vi "System Test.vi"(11 "Data Folder":path) -> ()   [LabVIEW 2020]
uses:
  epl-vi-lib/Signal Synthesis VIs/Controls/Multichannel (Full)/Multichannel (Full).xctl
  epl-vi-lib/Utility VIs/Type Defs/Speaker ring.ctl
  <vilib>/Analysis/5stat.llb/RMS (DBL).vi
  epl-vi-lib/Utility VIs/Math VIs/Linear to dB (scalar).vi
  epl-vi-lib/PXI DAQ VIs/DAQ Engine VIs/PXI Globals.vi
  epl-vi-lib/Signal Synthesis VIs/Waveform VIs/Noise VIs/Noise-Globals.vi
  <vilib>/Analysis/NI_AALPro.lvlib
panel:
  in  "Trigger":bool caption="Generate trigger"
  out "exit signal":bool
  out "Cal mic index":i32
  in  "Cal mic":T1={"dB SPL"=0.0, "Mode"=enum."Avg", "Mic gain (dB)"=40.0, "Sensitivity (dB V/SPL)"=-160.0} {"dB SPL" format="%.1f"}
  in  "input selections":i32[](array[numeric])
  in  "Start":bool
  out "Abort":bool
  out "AI Chans":i32[](array[numeric])
  out "AO Chans":i32[](array[numeric])
  out "AI graph":dbl[][](graph)
  in  "AO Sampling Rate (Hz)":dbl=100000.0
  in  "AI Sampling Rate (Hz)":dbl=25000.0
  in  "Total Duration (ms)":dbl=500.0
  out "Stimulus graph":dbl[][](graph)
  in  "Input Channels":i32(listbox)
  in  "Update":bool
  in  "Stop":bool
  in  "Use mapping":bool=TRUE
  in  "Quit":bool
  in  "Stimulus Channels":T2[](xcontrol)
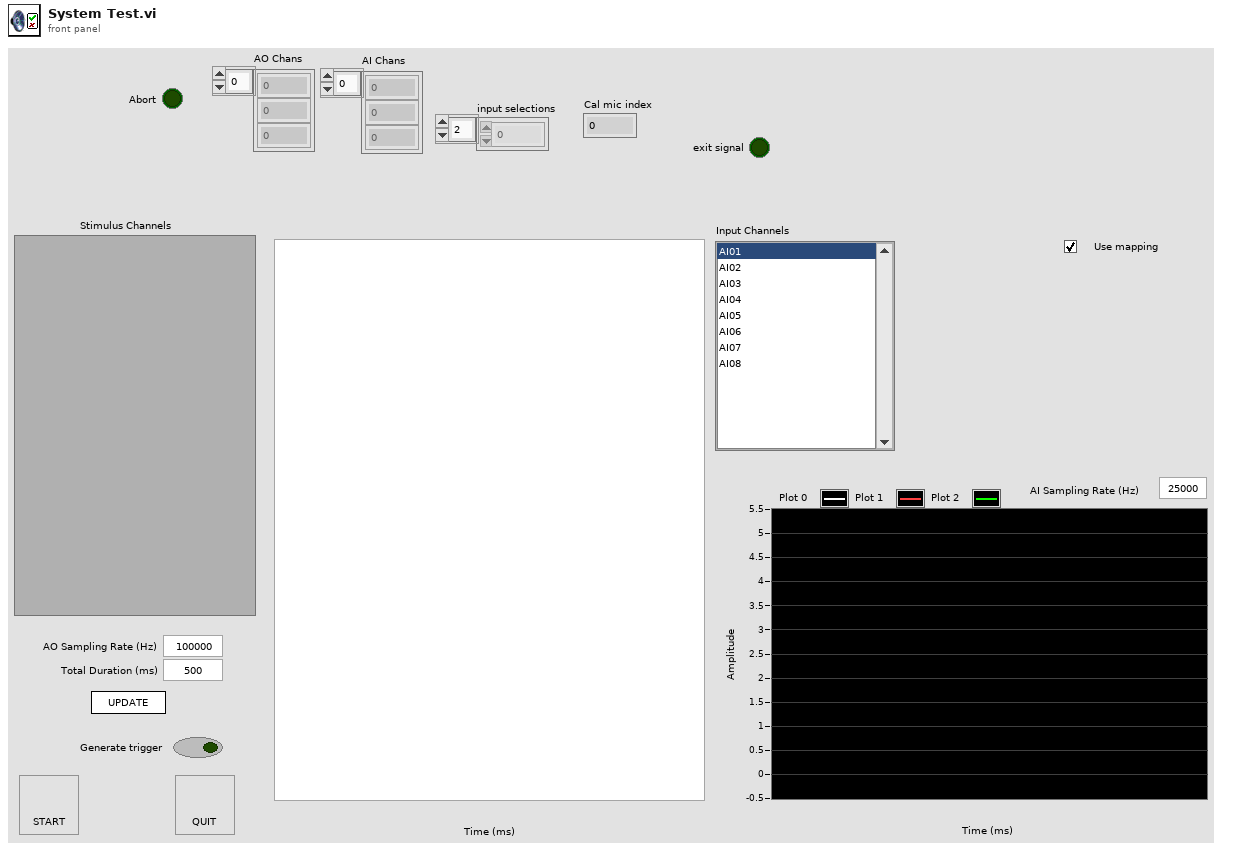
[diagram p1: front panel]
types:
  T1 = cluster{"dB SPL":dbl, "Mode":enum16{"Avg", "Peak"}, "Mic gain (dB)":dbl, "Sensitivity (dB V/SPL)":dbl}
  T2 = typedef "Stimulus Channel (Full).xctl/Full Stimulus Channel Data.ctl" = cluster{"Waveform":T3, "Filter":T20, "Burst":T22, "Level":T23, "Name":string, "Advanced":T25, "SAM":T26}
  T3 = typedef "Waveform XCtl.xctl/Waveform Data.ctl" = cluster{"Type":T4, "Tone":T5, "Pulse Train":T6, "Noise":T9, "File":T10, "FMSweep":T11, "Chirp Train":T12, "Complex Tone":cluster{"Params":T14, "Data":T16}, "Moving Ripple":T17}
  T4 = typedef "Waveform Enum.ctl" = enum16{"OFF", "Tone", "Noise", "Pulse Train", "File", "FM Sweep", "Chirp Train", "Complex Tone", "FM Tone", "Moving Ripple"}
  T5 = typedef "Tone Params.ctl" = cluster{"Frequency (kHz)":dbl, "Last Freq":dbl, "Last Phase":dbl}
  T6 = typedef "Pulse Train Params.ctl" = cluster{"Pulse width (us)":dbl, "Pulse rate (Hz)":dbl, "Gap (ms)":dbl, "Polarity":T7, "PT State":T8, "Asynch":bool}
  T7 = typedef "Pulse Polarity.ctl" = enum16{"POS", "NEG", "POS-NEG", "NEG-POS"}
  T8 = typedef "PT-Continuous State.ctl" = cluster{"Template":dbl[], "Nperiod":i32, "Index":i32, "Pulse Rate (Hz)":dbl, "Phase (cycles)":dbl, "Noff":i32}
  T9 = typedef "Noise Params.ctl" = cluster{"InvFilt":bool, "Noise":dbl[], "CurPt":i32, "Aweight":bool, "Seed":i32, "afile":path}
  T10 = typedef "StimFile-Params.ctl" = cluster{"Filename":path, "Signal":dbl[], "Channel":i32, "stream":bool, "offset":i32, "nreps":i32, "loops":i32, "Randomize":bool, "order":i32[], "Seed":i32, "Tokens":i32}
  T11 = typedef "FM Sweep Params.ctl" = cluster{"Rate (oct/s)":dbl, "Fmin (Hz)":dbl, "Fmax (Hz)":dbl, "Ramp (ms)":dbl, "Linear":bool}
  T12 = typedef "Chirp Train.ctl" = cluster{"Params":T13, "Data":cluster{"WF":dbl[]}}
  T13 = typedef "Chirp Train Params.ctl" = cluster{"Fmin (kHz)":dbl, "Fmax (kHz)":dbl, "Compensate":bool, "Duration (ms)":dbl}
  T14 = typedef "CT-Params.ctl" = cluster{"F0 (Hz)":dbl, "Band":cluster{"Flow (Hz)":dbl, "Fhigh (Hz)":dbl}, "Phase":T15, "Min F0 (Hz)":dbl, "Max F0 (Hz)":dbl, "ContinRandPhase":bool, "Max peak factor":dbl, "Max mod depth":dbl, "MinHarmNum":i32, "MaxHarmNum":i32, "Level Mode":enum16{"per component", "overall rms"}, "% jitter":dbl}
  T15 = typedef "CT-Phase Enum.ctl" = enum16{"Cosine", "Random", "Alternating"}
  T16 = typedef "CT-Runtime Data.ctl" = cluster{"Ncomp":i32, "MinHarm":i32, "Phase":dbl[], "Amplitude":dbl[], "Npts/frame":i32, "Last F0":dbl, "Fmin":dbl, "Fmax":dbl, "Lslope":dbl, "randphase":bool, "overall rms":bool, "fmult":dbl[], "jittered":bool}
  T17 = typedef "Moving Ripple.ctl" = cluster{"Params":T18, "Data":T19}
  T18 = typedef "Moving Ripple.Params.ctl" = cluster{"Fmin":dbl, "Fmax":dbl, "Density":dbl, "Velocity":dbl, "Depth":dbl, "Phase":dbl, "Comp/oct":i32}
  T19 = typedef "Moving Ripple.Data.ctl" = cluster{"Freq":dbl[], "A":dbl[], "phase":dbl[], "Phase":dbl}
  T20 = typedef "Advanced Filter XCtl.xctl/Filter Data.ctl" = cluster{"Type":enum16{"Lowpass", "Highpass", "Bandpass", "Bandstop", "OFF"}, "CF (kHz)":dbl, "BW (kHz)":dbl, "Cascade":bool, "Quadrature":bool, "Scale Factor":dbl, "Stages":cluster{"IIR Filter":cluster{"filter structure":enum32{"IIR 2nd Order", "IIR 4th Order"}, "Reverse Coefficients":dbl[], "Forward Coefficients":dbl[]}, "State":dbl[]}[], "Class":enum16{"Elliptic", "Butterworth"}, "Order":i32, "BWUnits":T21}
  T21 = typedef "Filter-Bandwidth Units.ctl" = enum16{"Linear", "Octaves", "Min-Max"}
  T22 = typedef "Burst Control.xctl/Burst Data.ctl" = cluster{"Active":bool, "Delay (ms)":dbl, "Duration (ms)":dbl, "Ramp (ms)":dbl, "Rate (Hz)":dbl, "Trepeat (ms)":dbl, "Repeat":bool}
  T23 = typedef "Level XCtl.xctl/Level Data.ctl" = cluster{"Level":dbl, "Units":T24, "Max":dbl, "Multiplier":dbl, "Cal File":path, "Cal":cluster{"Freq (Hz)":dbl[], "Mag (dB SPL)":dbl[], "Phase (deg)":dbl[]}}
  T24 = typedef "Level Units.ctl" = enum16{"dB atten", "dB SPL", "dB re 1 Vrms", "dB V/Hz½", "mW", "dB HL", "Volts", "dB mW"}
  T25 = typedef "Advanced Stimulus Options.xctl/Advanced Stimulus Options.ctl" = cluster{"Rep Mask":string, "AltPol":bool, "Var":string, "Expr":string, "Persist":bool}
  T26 = typedef "SAM Params.ctl" = cluster{"Active":bool, "Frequency (Hz)":dbl, "Depth":dbl, "Init Phase (cycles)":dbl, "phase (degrees)":dbl, "Asynch":bool}
  T27 = typedef "Multichannel (Full).xctl/Data.ctl" = T2[]
  T28 = typedef "Speaker ring.ctl" = enum16{"Right primary", "Right secondary", "Left primary", "Left secondary"}
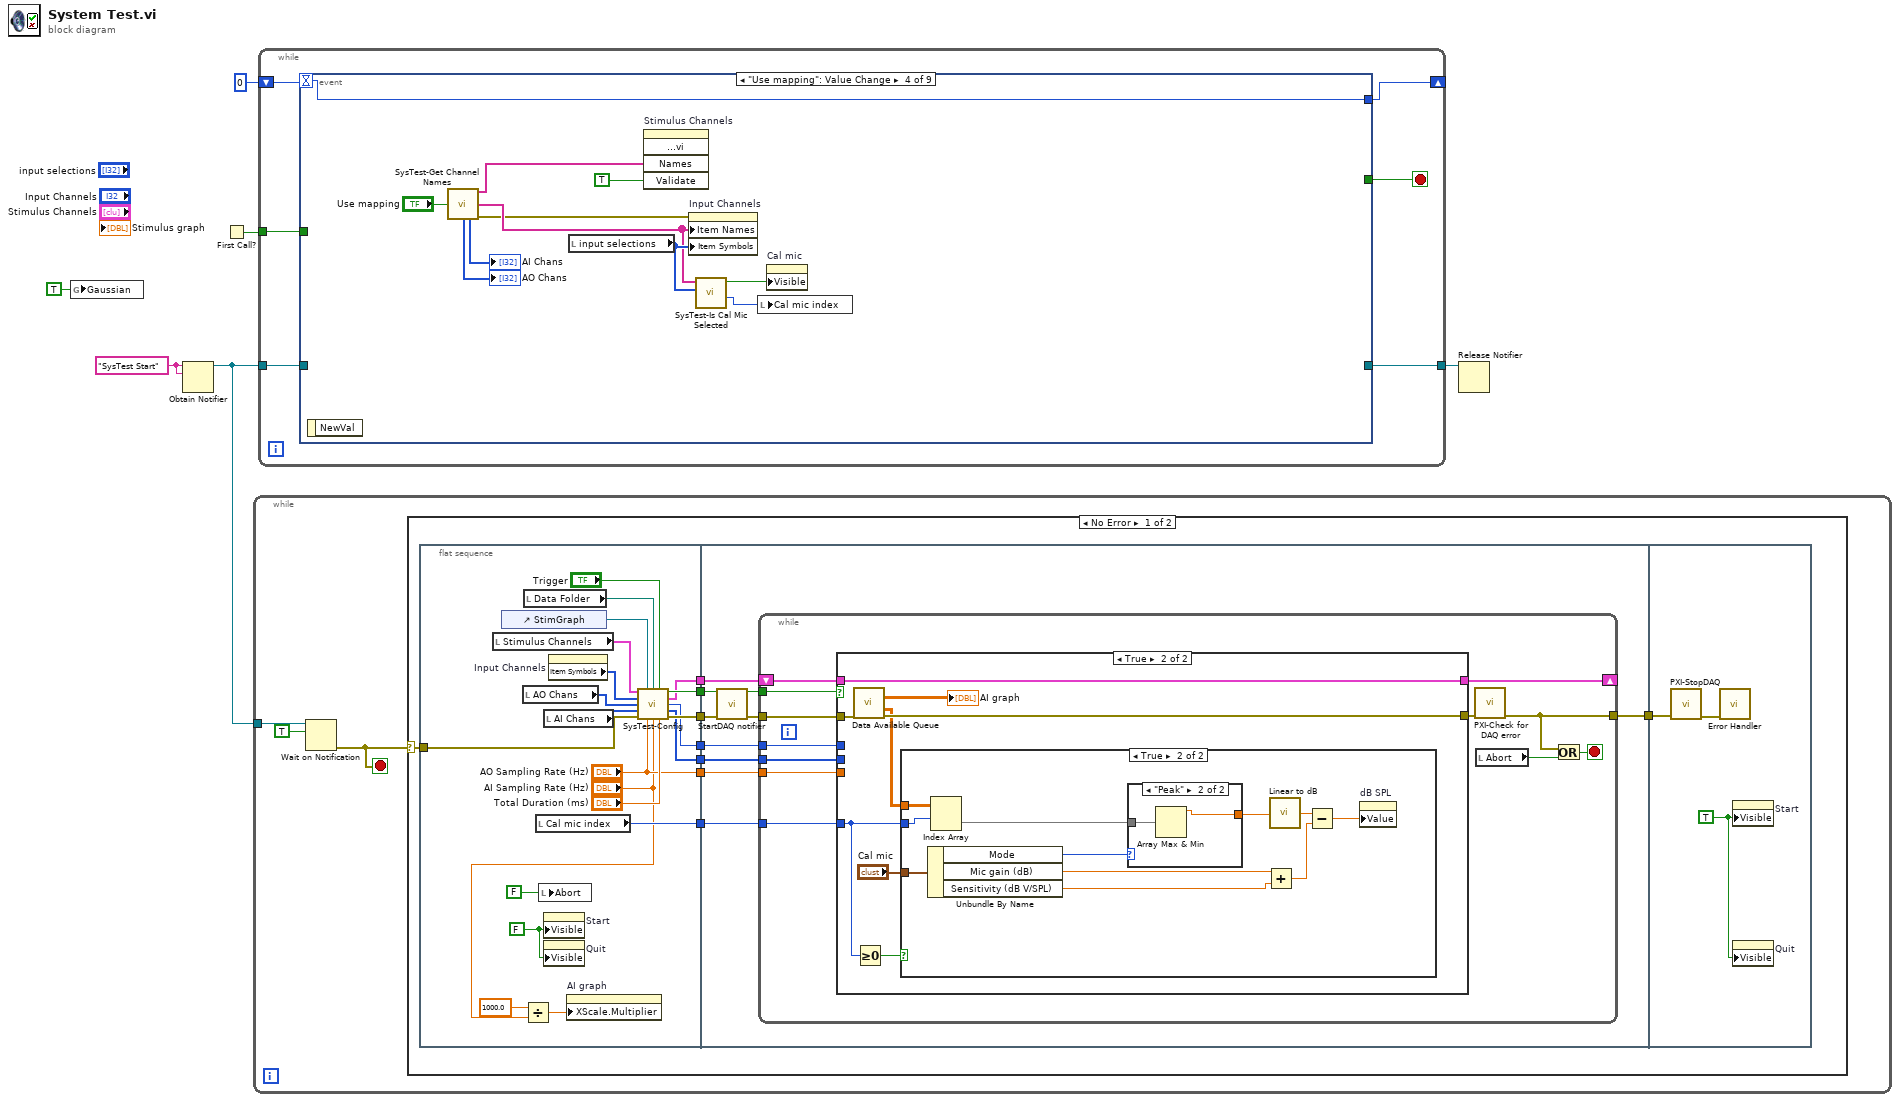
[diagram p0: block diagram]
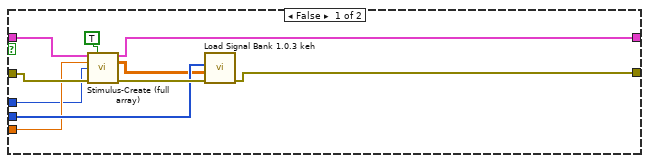
[diagram p2: hidden frame]
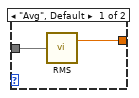
[diagram p4: hidden frame]
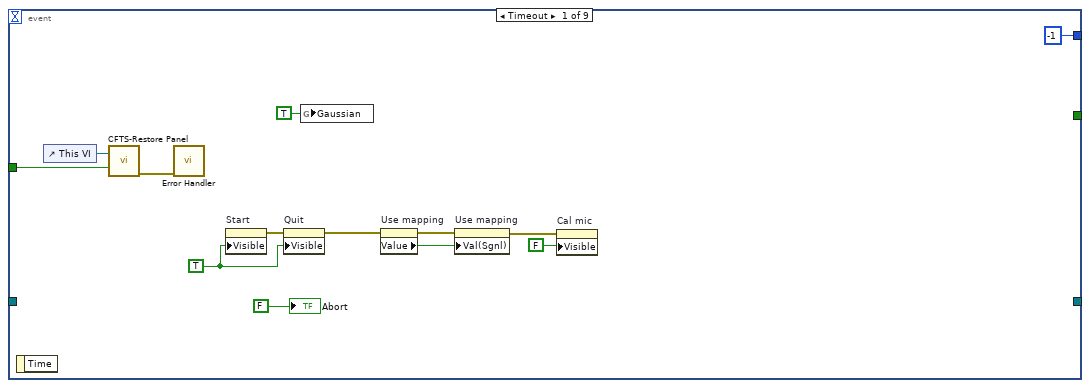
[diagram p6: hidden frame]
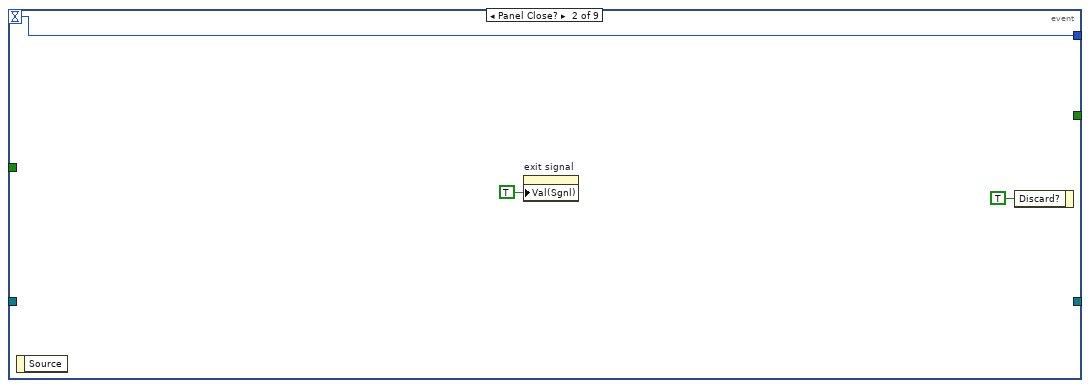
[diagram p7: hidden frame]
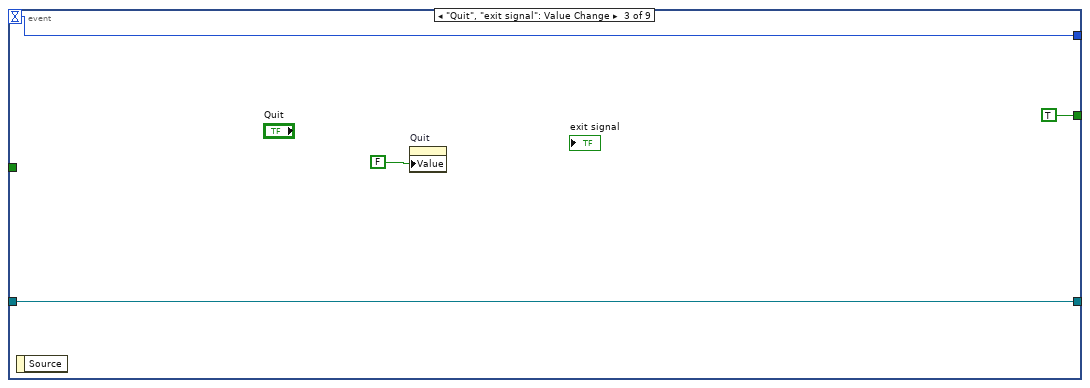
[diagram p8: hidden frame]
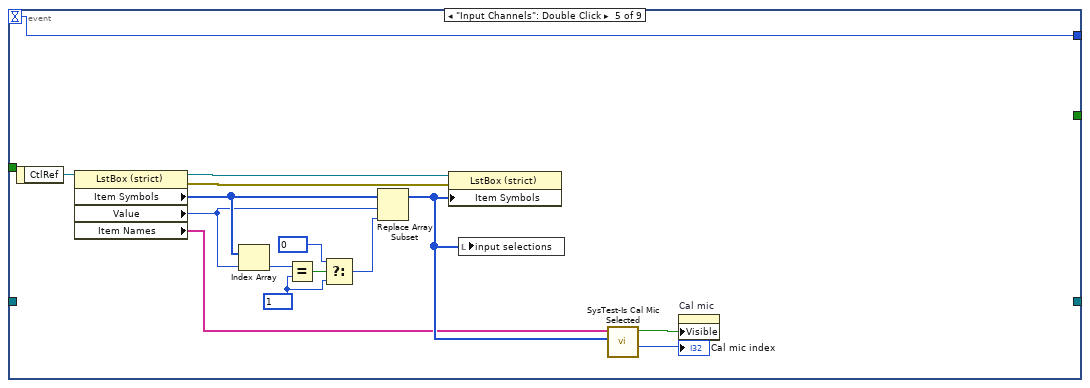
[diagram p9: hidden frame]
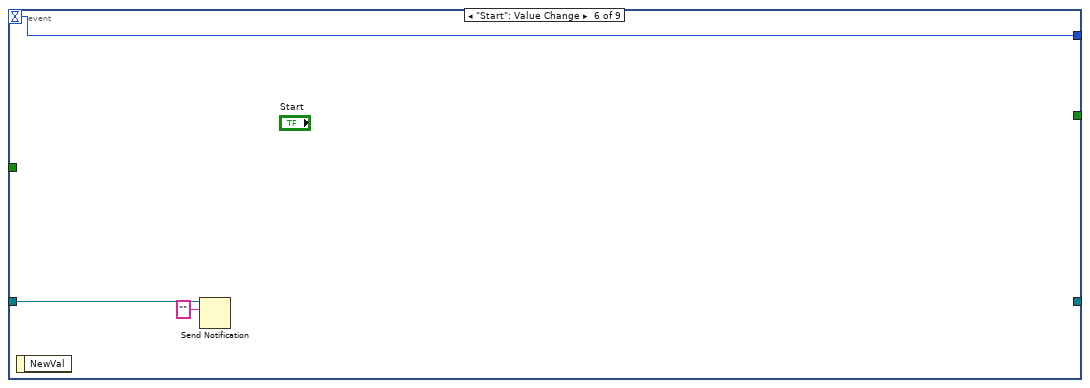
[diagram p10: hidden frame]
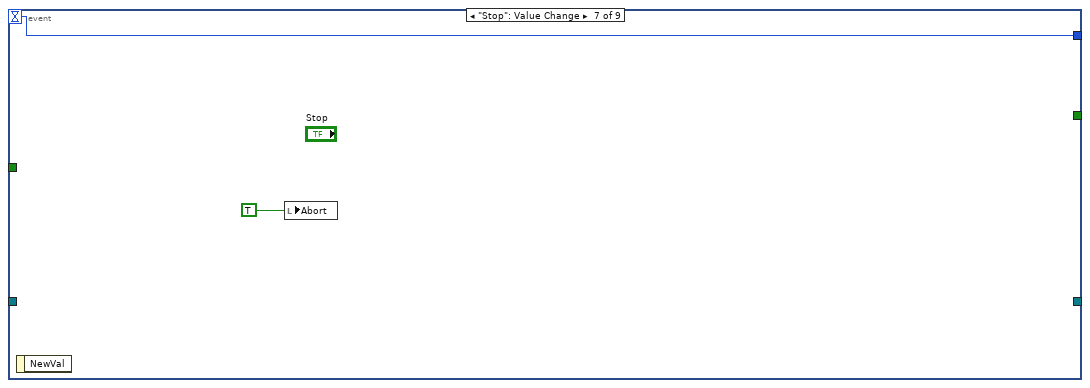
[diagram p11: hidden frame]
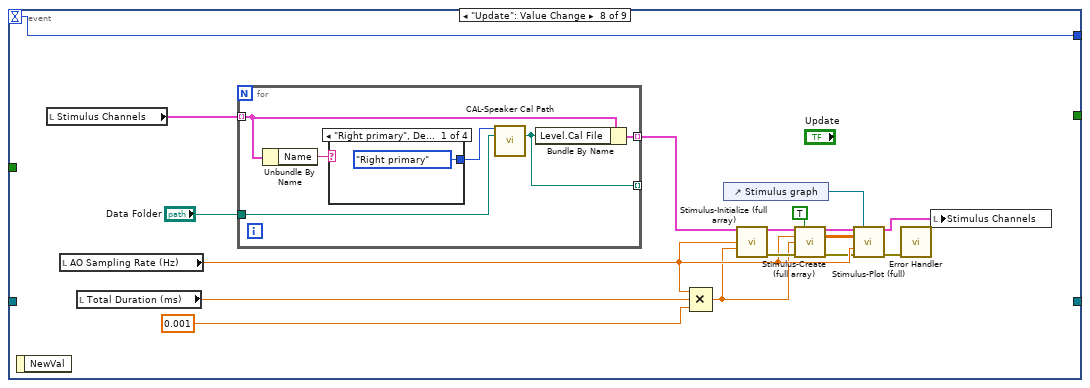
[diagram p12: hidden frame]
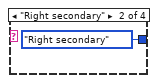
[diagram p13: hidden frame]
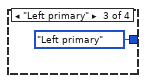
[diagram p14: hidden frame]
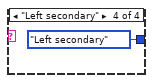
[diagram p15: hidden frame]
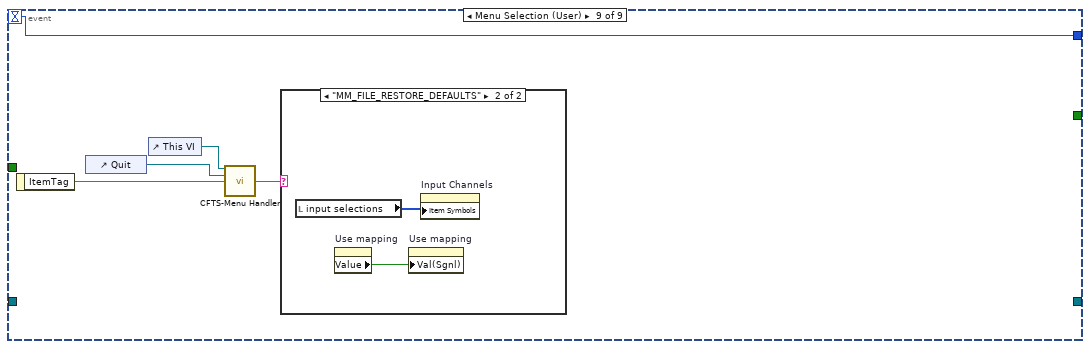
[diagram p16: hidden frame]
diagram:
  w5 = "SysTest Start" ("name (unnamed)")
  n1 = global write "Noise-Globals.vi" "Gaussian"(TRUE ("Gaussian")) -> ()
  n2 = Obtain Notifier(name (unnamed)=w5, notification data type=w5) -> (notifier out=w6:refnum<notifier>)  [unwired: 2 in, 2 out]
  n3 = First Call?() -> (First Call?: T/F=w2:bool)
  n4 = while {
    tunnel: w6 -> [w9]
    stop <- w7 stop-if-true
    n5 = Wait on Notification(notifier=w9, ignore previous (F)=TRUE) -> (error out=w7:errorcluster)  [unwired: 2 in, 3 out]
    n6 = case shown="No Error" w7 {
      selector: w7 -> [w18 _]
      frame No Error {
        n7 = flat-sequence {
          tunnel: w18 -> [w36]
          tunnel: [w34] -> w17
          tunnel: [w31] -> w15
          tunnel: [w27] -> w14
          tunnel: [w26] -> w13
          tunnel: ["AO Sampling Rate (Hz)"] -> w12
          tunnel: [w24] -> w11
          tunnel: [w23] -> w10
          tunnel: w17 -> [w48]
          tunnel: [w47] -> w16
          tunnel: w15 -> [w45]
          tunnel: w14 -> [w44]
          tunnel: w13 -> [w43]
          tunnel: w12 -> [w42]
          tunnel: w11 -> [w41]
          tunnel: w10 -> [w40]
          tunnel: w16 -> [w96]
          frame #0 {
            w30 = FALSE ("Visible")
            n8 = local read "Stimulus Channels"() -> (w39:T2[])
            n9 = control-ref of="StimGraph"() -> (w32:refnum<vi>)
            n10 = local read "AO Chans"() -> (w38:i32[])
            n11 = Divide(x=1000.0, y="AI Sampling Rate (Hz)") -> (x/y=w21:dbl)
            n12 = local read "Data Folder"() -> (w28:path)
            n13 = local read "Cal mic index"() -> (w27:i32)
            n14 = local write "Abort"(FALSE ("Global Abort")) -> ()
            n15 = local read "AI Chans"() -> (w37:i32[])
            n16 = property on="Start" class="Bool"("Visible"=w30) -> ()  [unwired: 2 in, 2 out]
            n17 = property on="Quit" class="Bool (strict)"("Visible"=w30) -> ()  [unwired: 2 in, 2 out]
            n18 = property on="Input Channels" class="LstBox (strict)"() -> ("Item Symbols"=w33:i32[])  [unwired: 2 in, 2 out]
            n19 = property on="AI graph" class="WFGraph (strict)"("XScale.Multiplier"=w21) -> ()  [unwired: 2 in, 2 out]
            n20 = call "SysTest-Config.vi"("AO Control"=w39, "Waveform Graph"=w32, "Data Folder"=w28, "Trigger"="Trigger", "Item Symbols"=w33, "AO Chans"=w38, "AI Chans"=w37, "error in (no error)"=w36, "AO Sampling Rate (Hz)"="AO Sampling Rate (Hz)", "AI Sampling Rate (Hz)"="AI Sampling Rate (Hz)", "Total Duration (ms)"="Total Duration (ms)") -> ("have AI?"=w31:bool, "StimChans Out"=w24:T27, "AO npts"=w23:i32, "AO Chans"=w26:i32[], "error out"=w34:errorcluster)
          }
          frame #1 {
            n21 = call "StartDAQ notifier.vi"("error in (no error)"=w48) -> ("error out"=w46:errorcluster)  [unwired: 6 in]
            n22 = while {
              tunnel: w46 -> [w60]
              tunnel: [w54] -> w47
              tunnel: w45 -> [w57]
              tunnel: w44 -> [w55]
              tunnel: w43 -> [w53]
              shift-right: [w52] -> _
              shift-left: w41 -> [w51]
              tunnel: w42 -> [w50]
              tunnel: w40 -> [w49]
              stop <- w59 stop-if-true
              n23 = case shown="True" w57 {
                tunnel: w60 -> [w70 w78]
                tunnel: [w62 w77] -> w58
                tunnel: w55 -> [_ w75]
                tunnel: w53 -> [w67 _]
                tunnel: [w65 w72] -> w52
                tunnel: w51 -> [w64 w72]
                tunnel: w50 -> [w63 _]
                tunnel: w49 -> [w61 _]
                frame False {
                  n24 = call "Stimulus-Create (full array).vi"("StimChan"=w64, "Apply multipliers? (F)"=TRUE ("Apply multipliers?"), "Sampling Rate (Hz)"=w63, "Npts"=w61, "error in (no error)"=w70) -> ("StimChan Out"=w65:T2[], "Waveform"=w66:dbl[][], "error out"=w68:errorcluster)  [unwired: 7 in, 1 out]
                  n25 = call "Load Signal Bank 1.0.3 keh.vi"("error in (no error)"=w68, "Input array"=w66, "Active AO Array"=w67) -> ("error out"=w62:errorcluster)  [unwired: 6 in, 2 out]
                }
                frame True {
                  n26 = call "Data Available Queue.vi"("error in (no error)"=w78) -> ("Waveform Graph"=→"AI graph":dbl[][], "AI Waveforms"=w74:dbl[][], "error out"=w77:errorcluster)  [unwired: 10 in, 2 out]
                  n27 = Greater Or Equal To 0?(x=w75) -> (x >= 0?=w76:bool)
                  n28 = case shown="True" w76 {
                    tunnel: w75 -> [_ w88]
                    tunnel: w74 -> [_ w89]
                    tunnel: "Cal mic" -> [_ w81]
                    frame False {
                    }
                    frame True {
                      n29 = Unbundle By Name(w81) -> ("Mode"=w80:enum16{"Avg", "Peak"}, "Mic gain (dB)"=w87:dbl, "Sensitivity (dB V/SPL)"=w86:dbl)
                      n30 = Index Array(array=w89, index (row)=w88) -> (element=w83:dbl[])  [unwired: 1 in]
                      n31 = case shown="\"Peak\"" w80 {
                        tunnel: [w91 w92] -> w84
                        tunnel: w83 -> [w90 w93]
                        frame "Avg", Default {
                          n32 = call-poly <vilib>:"RMS.vi"("X"=w90) -> ("rms value"=w91:dbl)  [unwired: 1 out]
                        }
                        frame "Peak" {
                          n33 = Array Max & Min(array=w93) -> (max value=w92:dbl)  [unwired: 3 out]
                        }
                      }
                      n34 = Add(x=w87, y=w86) -> (x+y=w82:dbl)
                      n35 = call-poly "Linear to dB.vi"("Linear"=w84) -> ("dB"=w85:dbl)
                      n36 = Subtract(x=w85, y=w82) -> (x-y=w79:dbl)
                      n37 = property on="dB SPL" class="DigNum (strict)"("Value"=w79) -> ()  [unwired: 2 in, 2 out]
                    }
                  }
                }
              }
              n38 = call "PXI-Check for DAQ error.vi"("error in (no error)"=w58) -> ("error out"=w54:errorcluster)  [unwired: 14 in]
              n39 = local read "Abort"() -> (w56:bool)
              n40 = Or(x=w54, y=w56) -> (x .or. y?=w59:bool)
            }
          }
          frame #2 {
            w94 = TRUE ("Visible")
            n41 = call "PXI-StopDAQ.vi"("error in (no error)"=w96) -> ("error out"=w95:errorcluster)  [unwired: 6 in]
            n42 = call "Error Handler.vi"("error in (no error)"=w95) -> ()  [unwired: 13 in, 2 out]
            n43 = property on="Start" class="Bool"("Visible"=w94) -> ()  [unwired: 2 in, 2 out]
            n44 = property on="Quit" class="Bool (strict)"("Visible"=w94) -> ()  [unwired: 2 in, 2 out]
          }
        }
      }
      frame Error {
      }
    }
  }
  n45 = while {
    tunnel: w6 -> [w101]
    tunnel: [w100] -> w4
    shift-right: [w98] -> _
    shift-left: 0 -> [w99]
    tunnel: w2 -> [w97]
    stop <- w102 stop-if-true
    n46 = event shown="[3] \"Use mapping\": Value Change" {
      selector: _ -> [_ _ _ _ _ _ _ _ _]
      dyn-events: _ -> [_ _ _ _ _ _ _ _ _]
      timeout: w99 -> [_ w116 w120 w132 w138 w149 w152 w170 w182]
      tunnel: [_ _ TRUE _ _ _ _ _ _] -> w102
      tunnel: w101 -> [_ _ w121 _ _ w151 _ _ _]
      tunnel: [_ _ w121 _ _ _ _ _ _] -> w100
      tunnel: [-1 w116 w120 w132 w138 w149 w152 w170 w182] -> w98
      tunnel: w97 -> [w110 _ _ _ _ _ _ _ _]
      event Timeout {
        w113 = TRUE ("Visible")
        n47 = event-data() -> ()  [unwired: 1 in, 1 out]
        n48 = control-ref of="This VI"() -> (w111:refnum<vi>)
        n49 = call "CFTS-Restore Panel.vi"("VI refnum"=w111, "Restore?"=w110) -> ("error out"=w104:errorcluster)  [unwired: 12 in, 1 out]
        n50 = call "Error Handler.vi"("error in (no error)"=w104) -> ()  [unwired: 13 in, 2 out]
        n51 = property on="Start" class="Bool"("Visible"=w113) -> (error out=w114:errorcluster)  [unwired: 2 in, 1 out]
        n52 = property on="Quit" class="Bool (strict)"(error in=w114, "Visible"=w113) -> (error out=w109:errorcluster)  [unwired: 1 in, 1 out]
        n53 = global write "Noise-Globals.vi" "Gaussian"(TRUE ("Gaussian")) -> ()
        n54 = property on="Use mapping" class="Bool (strict)"(error in=w109) -> (error out=w107:errorcluster, "Value"=w108:bool)  [unwired: 1 in, 1 out]
        n55 = property on="Use mapping" class="Bool (strict)"(error in=w107, "Val(Sgnl)"=w108) -> (error out=w106:errorcluster)  [unwired: 1 in, 1 out]
        n56 = property on="Cal mic" class="Clust (strict)"(error in=w106, "Visible"=FALSE) -> ()  [unwired: 1 in, 2 out]
        "Abort" <- FALSE ("quitting?")
      }
      event Panel Close? {
        n57 = event-data() -> ()  [unwired: 1 in, 1 out]
        n58 = property on="exit signal" class="Bool (strict)"("Val(Sgnl)"=TRUE ("Value (Signaling)")) -> ()  [unwired: 2 in, 2 out]
        n59 = event-data("Discard?"=TRUE) -> ()  [unwired: 1 in, 1 out]
      }
      event "Quit", "exit signal": Value Change {
        n60 = event-data() -> ()  [unwired: 1 in, 1 out]
        n61 = property on="Quit" class="Bool (strict)"("Value"=FALSE) -> ()  [unwired: 2 in, 2 out]
      }
      event "Use mapping": Value Change {
        n62 = event-data() -> ()  [unwired: 1 in, 1 out]
        n63 = call "SysTest-Get Channel Names.vi"("Use channel mapping?"="Use mapping") -> ("AO Names"=w124:string[], "AI Names"=w128:string[], "AO Chans"=→"AO Chans":i32[], "AI Chans"=→"AI Chans":i32[], "error out"=w125:errorcluster)  [unwired: 10 in]
        n64 = local read "input selections"() -> (w129:i32[])
        n65 = invoke on="Stimulus Channels" class="Multichannel (Full) (strict)" method="Set Channel Names.vi"("Names"=w124, "Validate"=TRUE) -> ()  [unwired: 3 in, 5 out]
        n66 = property on="Input Channels" class="LstBox (strict)"(error in=w125, "Item Names"=w128, "Item Symbols"=w129) -> ()  [unwired: 1 in, 2 out]
        n67 = call "SysTest-Is Cal Mic Selected.vi"("input selections"=w129, "AI Names"=w128) -> ("Cal mic index"=w126:i32, "Cal mic selected?"=w127:bool)  [unwired: 8 in]
        n68 = local write "Cal mic index"(w126) -> ()
        n69 = property on="Cal mic" class="Clust (strict)"("Visible"=w127) -> ()  [unwired: 2 in, 2 out]
      }
      event "Input Channels": Double Click {
        w140 = 1
        n70 = event-data() -> ("CtlRef"=w148:refnum<vi>)  [unwired: 1 in]
        n71 = property class="LstBox (strict)"(reference=w148) -> (reference out=w142:refnum<vi>, error out=w141:errorcluster, "Item Symbols"=w144:i32[], "Value"=w143:i32, "Item Names"=w135:string[])  [unwired: 1 in]
        n72 = Index Array(array=w144, index=w143) -> (element=w147:i32)
        n73 = Equal?(x=w147, y=w140) -> (x = y?=w146:bool)
        n74 = Select(t=0, s=w146, f=w140) -> (s? t:f=w145:i32)
        n75 = Replace Array Subset(array=w144, new element=w145, index=w143) -> (w136:i32[])
        n76 = property class="LstBox (strict)"(reference=w142, error in=w141, "Item Symbols"=w136) -> ()  [unwired: 2 out]
        n77 = local write "input selections"(w136) -> ()
        n78 = call "SysTest-Is Cal Mic Selected.vi"("input selections"=w136, "AI Names"=w135) -> ("Cal mic index"=→"Cal mic index":i32, "Cal mic selected?"=w137:bool)  [unwired: 8 in]
        n79 = property on="Cal mic" class="Clust (strict)"("Visible"=w137) -> ()  [unwired: 2 in, 2 out]
      }
      event "Start": Value Change {
        n80 = event-data() -> ()  [unwired: 1 in, 1 out]
        n81 = Send Notification(notification="", notifier=w151) -> ()  [unwired: 1 in, 2 out]
      }
      event "Stop": Value Change {
        n82 = event-data() -> ()  [unwired: 1 in, 1 out]
        n83 = local write "Abort"(TRUE ("Global Abort")) -> ()
      }
      event "Update": Value Change {
        n84 = event-data() -> ()  [unwired: 1 in, 1 out]
        n85 = local read "Stimulus Channels"() -> (w157:T2[])
        n86 = local read "AO Sampling Rate (Hz)"() -> (w164:dbl)
        n87 = local read "Total Duration (ms)"() -> (w168:dbl)
        n88 = for {
          tunnel: w157 -> [w176] mode=indexing
          tunnel: "Data Folder" -> [w172]
          tunnel: [w175] -> w155 mode=indexing
          tunnel: [w171] -> _ mode=indexing
          n89 = Unbundle By Name(w176) -> ("Name"=w174:string)
          n90 = case shown="\"Right primary\", Default" w174 {
            tunnel: [Speaker_ring."Right primary" ("Speaker") Speaker_ring."Right secondary" ("Speaker") Speaker_ring."Left primary" ("Speaker") Speaker_ring."Left secondary" ("Speaker")] -> w173
            frame "Right primary", Default {
            }
            frame "Right secondary" {
            }
            frame "Left primary" {
            }
            frame "Left secondary" {
            }
          }
          n91 = call "CAL-Speaker Cal Path.vi"("Speaker"=w173, "Data Folder"=w172) -> ("Cal Path"=w171:path)  [unwired: 12 in, 1 out]
          n92 = Bundle By Name(cluster=w176, "Level.Cal File"=w171) -> (w175:T2)
        }
        n93 = Compound Arithmetic op=MULTIPLY(w164, w168, 0.001 ("value")) -> (w154:dbl)
        n94 = control-ref of="Stimulus graph"() -> (w169:refnum<vi>)
        n95 = call "Stimulus-Initialize (full array).vi"("StimChans"=w155, "Sampling rate (Hz)"=w164, "Npts"=w154) -> ("StimChans Out"=w159:T2[], "error out"=w165:errorcluster)  [unwired: 10 in, 1 out]
        n96 = call "Stimulus-Create (full array).vi"("StimChan"=w159, "Apply multipliers? (F)"=TRUE ("Apply multipliers?"), "Sampling Rate (Hz)"=w164, "Npts"=w154, "error in (no error)"=w165) -> ("StimChan Out"=w161:T2[], "Waveform"=w162:dbl[][], "error out"=w163:errorcluster)  [unwired: 7 in, 1 out]
        n97 = call "Stimulus-Plot (full).vi"("AO Control"=w161, "Waveform Graph"=w169, "Array"=w162, "Sampling Rate (Hz)"=w164, "error in (no error)"=w163) -> ("AO Control out"=w158:T2[], "error out"=w166:errorcluster)  [unwired: 8 in, 1 out]
        n98 = call "Error Handler.vi"("error in (no error)"=w166) -> ()  [unwired: 13 in, 2 out]
        n99 = local write "Stimulus Channels"(w158) -> ()
      }
      event Menu Selection (User) {
        n100 = event-data() -> ("ItemTag"=w184:string)  [unwired: 1 in]
        n101 = control-ref of="Quit"() -> (w183:refnum<vi>)
        n102 = control-ref of="This VI"() -> (w185:refnum<vi>)
        n103 = call "CFTS-Menu Handler.vi"("VI Refnum"=w185, "Return Refnum"=w183, "ItemTag"=w184) -> ("ItemTag out"=w181:string)  [unwired: 11 in, 1 out]
        n104 = case shown="\"MM_FILE_RESTORE_DEFAULTS\"" w181 {
          frame "False", Default {
          }
          frame "MM_FILE_RESTORE_DEFAULTS" {
            n105 = local read "input selections"() -> (w187:i32[])
            n106 = property on="Use mapping" class="Bool (strict)"() -> ("Value"=w186:bool)  [unwired: 2 in, 2 out]
            n107 = property on="Use mapping" class="Bool (strict)"("Val(Sgnl)"=w186) -> ()  [unwired: 2 in, 2 out]
            n108 = property on="Input Channels" class="LstBox (strict)"("Item Symbols"=w187) -> ()  [unwired: 2 in, 2 out]
          }
        }
      }
    }
  }
  n109 = Release Notifier(notifier=w4) -> ()  [unwired: 2 in, 3 out]
